vi "Data Analysis VI.vi"() -> ()   [LabVIEW 2022 SP3]
uses:
  0d05760f-8841-43ce-bf7e-76eea4fe5a42.vi
  <vilib>/Utility/file.llb/Read Delimited Spreadsheet (string).vi
  <vilib>/addons/Time Series Analysis/Statistical Analysis.llb/TSA Confidence Limits (Array).vi
  <vilib>/addons/Time Series Analysis/Statistical Analysis.llb/TSA Mean (Array).vi
  <vilib>/addons/Time Series Analysis/Series Preprocess.llb/TSA Moving Average (Array).vi
  <vilib>/addons/Time Series Analysis/Statistical Analysis.llb/TSA Vector Deviation and Variance (Waveform).vi
  <vilib>/addons/_Advanced Signal Processing/NI_AdvSigProcTSA.lvlib
  <vilib>/gmath/NI_Gmath.lvlib
  <vilib>/addons/Time Series Analysis/Series Preprocess.llb/TSA Moving Average (Waveform).vi
panel:
  in  "Which Days to Plot?":cluster{"Boolean":bool, "String":string}[](array[cluster])=[{"Boolean"=FALSE, "String"="Day 1"}, {"Boolean"=FALSE, "String"="Day 2"}, {"Boolean"=FALSE, "String"="Day 3"}, {"Boolean"=FALSE, "String"="Day 4"}, {"Boolean"=FALSE, "String"="Day 5"}]
  in  "What to Plot?":u16(ring) items=["X-Ray Tests (3 Days)", "Further Tests (5 Days)"]
  out "Calculate Temperature Change from Power Density - using formula described in Ekin.":cluster{dbl[], dbl[]}(graph)
  out "Voltage @ 1st Current Increment":cluster{dbl[], dbl[]}(graph)
  out "Dosage vs Ic":cluster{dbl[], dbl[]}(graph)
  out "decimated array 2":dbl[](array[numeric])
  out "decimated array":dbl[](array[numeric])
  out "Temperature Normaliser":cluster{dbl[], dbl[]}[](graph)
  out "Ic Power Law vs Time (COMPARE) 2":cluster{"Relative Times":dbl[], dbl[]}(graph)
  out "Array 3":path[](array[path])
  out "Array 2":path[](array[path])
  out "x = y?":bool
  out "Temperature vs Ic":T1(graph)
  in  "TempInterpolate Method":i32(ring)=2 items=["nearest", "linear", "spline", "cubic Hermite", "Lagrange"]
  in  "TempInterpolate Reverse Method":i32(ring)=2 items=["nearest", "linear", "spline", "cubic Hermite", "Lagrange"]
  out "Ic Temperature Curve of THEVA HTS Tape 2":cluster{"Temp Data":dbl[], "Ic Data":dbl[]}[](graph)
  out "NumPlots":i32
  out "Relative Times NaN'd":dbl[](array[numeric])
  out "Relative Times":dbl[](array[numeric])
  out "Dosage Characteristics":cluster{dbl[], dbl[]}[](graph)
  in  "Plot?":bool[](array[boolean])
  out "Concatenated Ic vs Time":cluster{dbl[], dbl[]}[](graph)
  out "Ic Power Law vs Time (COMPARE)":cluster{dbl[], dbl[]}[](graph)
  out "Historical Data 2":cluster{"Array":dbl[], "Array":dbl[]}[](graph)
  in  "(Baseline 1st)Shifted":dbl[](array[numeric])=[-200.4, -200.5] format="%#_13g"
  out "Expected Ic Fluctuation due to specified temperature range (A)":dbl[](array[numeric])
  out "percentage change":dbl[](array[numeric])
  out "Ic Temperature Curve of THEVA HTS Tape":cluster{"all rows":dbl[], "all rows":dbl[]}[](graph)
  out "Ic and Temperature vs Time":cluster{dbl[], dbl[]}[](graph)
  in  "length":i32=100
  in  "index":i32=20
  out "LogLog":cluster{dbl[], dbl[]}[](graph)
  out "error out":errorcluster
  out "Experimental Ic vs Temperature Corrected Ic":cluster{dbl[], dbl[]}[](graph)
  out "Absolute Ic Fluctuation":cluster{dbl[], dbl[]}(graph)
  out "Mean Run Temperature vs Time":cluster{dbl[], dbl[]}(graph)
  in  "Selected":dbl=10.0
  out "Different Model Comparisons for Selected Run":cluster{"Array":dbl[], "Array":dbl[]}[](graph)
  out "Compare Different Models vs TIME/DOSAGE":cluster{dbl[], dbl[]}[](graph)
  out "Total Dose over Measurement time (kGy)":dbl
  out "Maximum Dosage Rate (kGy/h)":dbl
  in  "Estimated Dose Rate 12cm from tube (Gy/s)":dbl=23.7
  out "Time vs Temperature":cluster{dbl[], dbl[]}(graph)
  out "Number of Runs":dbl
  out "Experiment Description":variant
  out "current time":timestamp
  in  "Array":path[](array[path])=[path "C:/Users/kumarr3/OneDrive - Victoria University of Wellington - STAFF/Documents/DataFiles/Xray runs/xray_FIRSTRUN", path "C:/Users/kumarr3/OneDrive - Victoria University of Wellington - STAFF/Documents/DataFiles/Xray runs/xray_secondrun_1902", path "C:/Users/kumarr3/OneDrive - Victoria University of Wellington - STAFF/Documents/DataFiles/Xray runs/xray_thirdrun_morning_2102", path "C:/Users/kumarr3/OneDrive - Victoria University of Wellington - STAFF/Documents/DataFiles/Copper Tests/Thursday_mixingtesting_01_voltmeter_alreadyON", path "C:/Users/kumarr3/OneDrive - Victoria University of Wellington - STAFF/Documents/DataFiles/Copper Tests/Thursday_mixingtesting_01_voltmeter_alreadyON", path "C:/Users/kumarr3/OneDrive - Victoria University of Wellington - STAFF/Documents/DataFiles/Copper Tests/Friday_mixingtest_voltmeter_justturnedon", path "C:/Users/kumarr3/OneDrive - Victoria University of Wellington - STAFF/Documents/DataFiles/Copper Tests/Monday_mixingtest_voltmeterONallweekend", path "C:/Users/kumarr3/OneDrive - Victoria University of Wellington - STAFF/Documents/DataFiles/Copper Tests/Tuesday_bothmeters_onovernight"] caption="Load File Path or Directory"
  # "Data extracted from tdms file, plotted against TIME/DOSAGE"
  # "Temperature Correction Analysis"
  # "Loading Information"
  # "Temperature Interpolation"
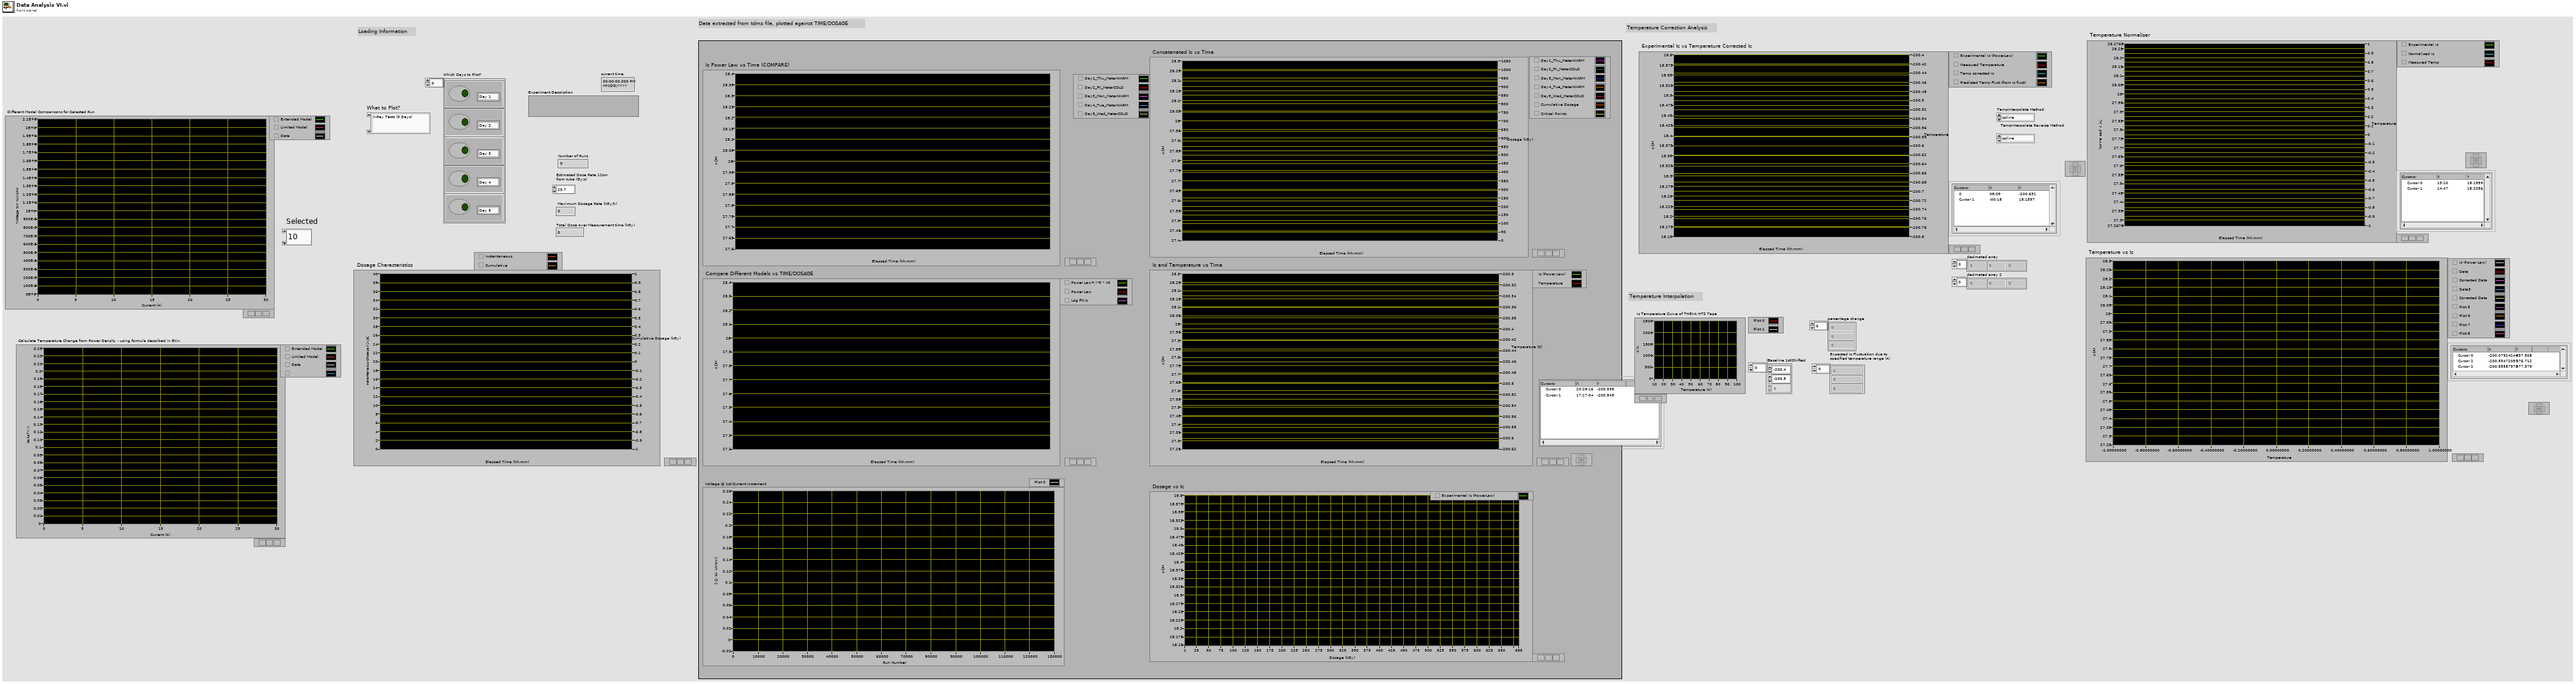
[diagram p1: front panel]
types:
  T1 = cluster{"Ic array (Power Law)":dbl[], "Mean Temp Array":dbl[]}[]
  T2 = cluster{"Dosage RelTimes":dbl[], "Cumul Dosages":dbl[], "Instantaneous Dosages":dbl[]}
  T3 = cluster{"Mean Temp Array":dbl[], "Lower Temp Array":dbl[], "Upper Temp Array":dbl[]}
  T4 = cluster{"Ic Array (Extnded)":dbl[], "Ic array (Power Law)":dbl[], "Relative Times":dbl[], "LogLog FIt":dbl[], "Absolute Ic Fluctuation":dbl[], "Temp Corrected Data":dbl[], "Upper Corrected":dbl[], "Lower Corrected":dbl[], "Smoothed Power Law":dbl[]}
  T5 = cluster{"I indexed":dbl[], "Best Linear Fit":dbl[]}
  T6 = cluster{"I indexed":dbl[], "Best Linear Fit":dbl[]}[]
  T7 = cluster{"Relative Times":dbl[], "Ic Array (Extnded)":dbl[]}
  T8 = cluster{"Relative Times":dbl[], "Ic Array (Extnded)":dbl[]}[]
  T9 = cluster{"Instant. Dos. Times":dbl[], "Instant. Dosages":dbl[]}
  T10 = cluster{"Cumul Dos. Times":dbl[], "Cumul Dosages":dbl[]}
  T11 = cluster{"Cumul Dos. Times":dbl[], "Cumul Dosages":dbl[]}[]
  T12 = cluster{"Critical Times":dbl[], "Critical Dosages":dbl[]}
  T13 = cluster{"Mean Temp Array":dbl[], "Ic array (Power Law)":dbl[]}
  T14 = cluster{"Predicted Temp (C)":dbl[], "xi used":dbl[]}
  T15 = cluster{"Relative Times NaN'd":dbl[], "Corrected Ic":dbl[]}
  T16 = cluster{"Predicted Temp (C)":dbl[], "xi used":dbl[]}[]
  T17 = cluster{"Mean Temp Array":dbl[], "Corrected Ic":dbl[]}[]
  T18 = cluster{"Relative Times NaN'd":dbl[], "Predicted Temp (C)":dbl[]}
  T19 = cluster{"Critical Times":dbl[], "Critical Dosages":dbl[]}[]
  T20 = cluster{"Relative Times NaN'd":dbl[], "Predicted Temp (C)":dbl[]}[]
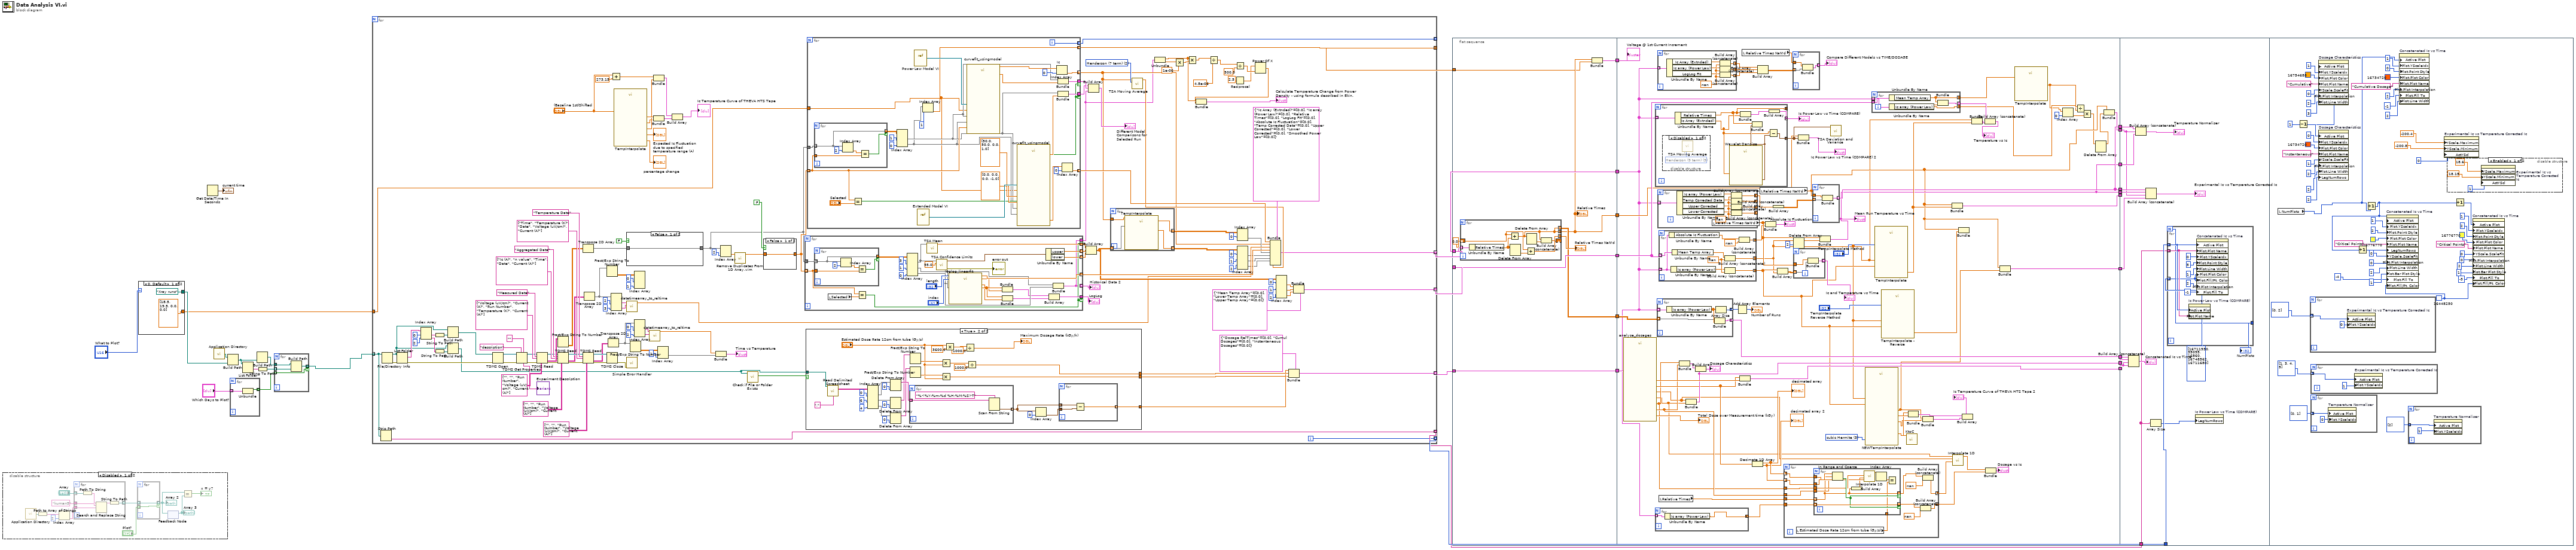
[diagram p0: block diagram]
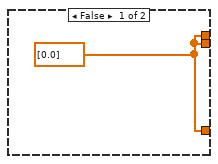
[diagram p2: hidden frame]
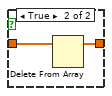
[diagram p3: hidden frame]
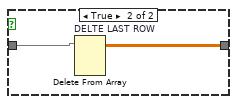
[diagram p4: hidden frame]
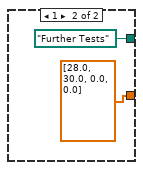
[diagram p6: hidden frame]
diagram:
  n1 = disable-structure shown="Disabled" {
    frame Disabled {
      n2 = call <vilib>:"Application Directory.vi"() -> ("Application Directory"=w41:path)
      n3 = Path to Array of Strings(0:w41) -> (2:w42:string[])  [unwired: 1 out]
      n4 = Index Array(array=w42, index=2) -> (element=w43:string)
      n5 = for {
        tunnel: "Array" -> [w51] mode=indexing
        tunnel: w43 -> [w49]
        tunnel: "kumarr3" ("search string") -> [w48]
        tunnel: [w46] -> w45 mode=indexing
        n6 = Path To String(path=w51) -> (string=w50:string)
        n7 = Search and Replace String(input string=w50, search string=w48, replace string=w49) -> (result string=w47:string)  [unwired: 5 in, 3 out]
        n8 = String To Path(string=w47) -> (path=w46:path)
      }
      n9 = for {
        tunnel: [w53] -> w39 mode=indexing if=w52
        tunnel: w45 -> [w53] mode=indexing
        tunnel: "Plot?" -> [w52] mode=indexing
      }
      "Array 2" <- w39
      n10 = feedback #1() -> (w38:path[])  [unwired: 1 in]
      "Array 3" <- w38
      n11 = feedback-in #1(w39) -> ()
      n12 = Equal?(x=w39, y=w38) -> (x = y?=→"x = y?":bool)
    }
    frame Enabled {
    }
  }
  n13 = case shown="0, Default" "What to Plot?" {
    tunnel: [path "Xray runs" path "Further Tests"] -> w9
    tunnel: [dbl[] [18.5, 19.5, 0.0, 0.0] dbl[] [28.0, 30.0, 0.0, 0.0]] -> w1
    frame 0, Default {
    }
    frame 1 {
    }
  }
  n14 = Get Date/Time In Seconds() -> (seconds since 1Jan1904=→"current time":timestamp)
  n15 = call <vilib>:"Application Directory.vi"() -> ("Application Directory"=w8:path)
  n16 = Build Path(base path=w8, name or relative path=w9) -> (appended path=w6:path)
  n17 = for {
    tunnel: "Which Days to Plot?" -> [w59] mode=indexing
    tunnel: [w58] -> w4 mode=indexing
    n18 = Unbundle(w59) -> ("Boolean"=w58:bool)  [unwired: 1 out]
  }
  n19 = List Folder(path=w6) -> (folder names=w7:string[])  [unwired: 3 in, 3 out]
  n20 = Build Path(name or relative path=w6) -> (appended path=w3:path)  [unwired: 1 in]
  n21 = String To Path(string=w7) -> (path=w5:path[])
  n22 = for {
    tunnel: [w60] -> w2 mode=indexing if=w63
    tunnel: w5 -> [w61] mode=indexing
    tunnel: w4 -> [w63] mode=indexing
    tunnel: w3 -> [w62]
    n23 = Build Path(base path=w62, name or relative path=w61) -> (appended path=w60:path)
  }
  n24 = for {
    tunnel: w2 -> [w140] mode=indexing
    tunnel: [w85] -> w22 mode=indexing
    tunnel: [w84] -> w21 mode=indexing
    tunnel: [w83] -> w20 mode=indexing
    tunnel: [w107] -> w19 mode=indexing
    tunnel: [w106] -> w18 mode=indexing
    tunnel: [w80] -> _ mode=indexing
    tunnel: [w79] -> w13 mode=concatenating
    tunnel: w1 -> [w64]
    i -> [w107]
    w97 = 2 items=["Spencer (15 term)"=1, "Henderson (7 term)"=2, "Henderson (9 term)"=3, "Henderson (13 term)"=4, "Henderson (23 term)"=5] ("method")
    n25 = Strip Path(path=w140) -> (name=w106:string)  [unwired: 1 out]
    n26 = File/Directory Info(path=w140) -> (path out=w113:path, error out=w200:errorcluster)  [unwired: 1 in, 5 out]
    n27 = List Folder(path=w113, error in=w200) -> (filenames=w138:string[], error out=w198:errorcluster)  [unwired: 2 in, 2 out]
    n28 = Index Array(array=w138, index #1=0 ("index"), index #2=2 ("index")) -> (element #1=w139:string, element #2=w114:string)
    n29 = String To Path(string=w139) -> (path=w197:path)
    n30 = String To Path(string=w114) -> (path=w112:path)
    n31 = Build Path(base path=w113, name or relative path=w197) -> (appended path=w157:path)
    n32 = Build Path(base path=w113, name or relative path=w112) -> (appended path=w81:path)
    n33 = TDMS Open(8:w198, 11:w157) -> (0:w186:errorcluster, 3:w187:refnum<k34>)  [unwired: 5 in]
    n34 = TDMS Get Properties(5:"", 7:"description", 8:w186, 11:w187) -> (0:w184:errorcluster, 3:w185:refnum<k34>, 4:→"Experiment Description":string)  [unwired: 2 in, 3 out]
    n35 = TDMS Read(0:w185, 5:"Measured Data" ("group name in"), 7:string[] ["Voltage (uV/cm)", "Current (A)", "Run Number", "Temperature (K)", "Current (A)"] ("channel name(s) in (Untitled)"), 11:w184, 12:string[][] [["", "", "Run Number", "Voltage (uV/cm)", "Current (A)"]] ("channel name(s) in (Untitled)")) -> (4:w174:refnum<k34>, 10:w193:string[][], 15:w173:errorcluster)  [unwired: 3 in, 3 out]
    n36 = Fract/Exp String To Number(string=w193) -> (number=w156:dbl[][])  [unwired: 3 in, 1 out]
    n37 = TDMS Read(0:w174, 5:"Aggregated Data" ("group name in"), 7:string[] ["Ic (A)", "n value", "Time", "Date", "Current (A)"] ("channel name(s) in (Untitled)"), 11:w173, 12:string[][] [["", "", "Run Number", "Voltage (uV/cm)", "Current (A)"]] ("channel name(s) in (Untitled)")) -> (4:w172:refnum<k34>, 10:w166:string[][], 15:w171:errorcluster)  [unwired: 3 in, 3 out]
    n38 = TDMS Read(0:w172, 5:"Temperature Data" ("group name in"), 7:string[] ["Time", "Temperature (K)", "Date", "Voltage (uV/cm)", "Current (A)"] ("channel name(s) in (Untitled)"), 11:w171, 12:string[][] [["", "", "Run Number", "Voltage (uV/cm)", "Current (A)"]] ("channel name(s) in (Untitled)")) -> (4:w176:refnum<k34>, 10:w169:string[][], 15:w175:errorcluster)  [unwired: 3 in, 3 out]
    n39 = Transpose 2D Array(2D array=w156) -> (transposed array=w155:dbl[][])
    n40 = Transpose 2D Array(2D array=w166) -> (transposed array=w141:string[][])
    n41 = Fract/Exp String To Number(string=w141) -> (number=w165:dbl[][])  [unwired: 3 in, 1 out]
    n42 = TDMS Close(8:w175, 11:w176) -> (0:w180:errorcluster)  [unwired: 1 out]
    n43 = Transpose 2D Array(2D array=w169) -> (transposed array=w151:string[][])
    n44 = Add(x="(Baseline 1st)Shifted", y=273.15) -> (x+y=w91:dbl[])
    n45 = Index Array(array=w141, index (col) #1=2 ("disabled index (col)"), index (col) #2=3 ("index (col)")) -> (element #1=w150:string[], element #2=w122:string[])  [unwired: 2 in]
    n46 = call "TempInterpolate.vi"("(Baseline 1st) Shifted"="(Baseline 1st)Shifted") -> ("Temp Data"=w95:dbl[], "Ic Data"=w87:dbl[], "Ic Fluct (from baseline)"=→"Expected Ic Fluctuation due to specified temperature range (A)":dbl[], "percentage change"=→"percentage change":dbl[], "Raw Interpolated Ic"=w93:dbl[])  [unwired: 5 in, 1 out]
    n47 = case shown="False" FALSE {
      tunnel: w155 -> [w273 w275]
      tunnel: [w273 w274] -> w145
      frame False {
      }
      frame True {
        n48 = Delete From Array "DELTE LAST ROW"(array=w275) -> (array with subset deleted=w274:dbl[][])  [unwired: 3 in, 1 out]
      }
    }
    n49 = call "datetimearray_to_reltime.vi"("Date Array"=w122, "Time Array"=w150) -> ("Rel. time array"=w109:dbl[])  [unwired: 9 in]
    n50 = call <vilib>:"Simple Error Handler.vi"("error in (no error)"=w180) -> ()  [unwired: 2 in, 7 out]
    n51 = Fract/Exp String To Number(string=w151) -> (number=w168:dbl[][])  [unwired: 3 in, 1 out]
    n52 = Index Array(array=w165, index (col) #1=0 ("disabled index (col)"), index (col) #2=1 ("index (col)")) -> ()  [unwired: 2 in, 2 out]
    n53 = Index Array(array=w151, index (col) #1=0 ("disabled index (col)"), index (col) #2=2 ("index (col)")) -> (element #1=w154:string[], element #2=w119:string[])  [unwired: 2 in]
    n54 = call "datetimearray_to_reltime.vi"("Date Array"=w119, "Time Array"=w154) -> ("Rel. time array"=w153:dbl[])  [unwired: 9 in]
    n55 = Bundle(w91, "Raw Interpolated Ic"=w93) -> (w89:cluster{dbl[], "Raw Interpolated Ic":dbl[]})  [unwired: 1 in]
    n56 = Bundle("Temp Data"=w95, "Ic Data"=w87) -> (w88:cluster{"Temp Data":dbl[], "Ic Data":dbl[]})  [unwired: 1 in]
    n57 = Index Array(array=w168, index (col)=1 ("disabled index (col)")) -> (element=w161:dbl[])  [unwired: 1 in]
    n58 = Build Array(w89, w88) -> (→"Ic Temperature Curve of THEVA HTS Tape":cluster{"Temp Data":dbl[], "Ic Data":dbl[]}[])
    n59 = Bundle("Rel. time array"=w153, w161) -> (→"Time vs Temperature":cluster{"Rel. time array":dbl[], dbl[]})  [unwired: 1 in]
    n60 = Index Array(array=w145, index (col)=2 ("disabled index (col)")) -> (element=w160:dbl[])  [unwired: 1 in]
    n61 = call "Remove Duplicates From 1D Array.vim"("array"=w160) -> ("array with duplicates removed"=w148:dbl[])  [unwired: 10 in]
    n62 = call <vilib>:"Check if File or Folder Exists.vi"("path"=w81) -> ("file or folder exists?"=w82:bool)  [unwired: 8 in, 2 out]
    n63 = case shown="False" FALSE {
      tunnel: w148 -> [w270 w272]
      tunnel: [w270 w271] -> w146
      frame False {
      }
      frame True {
        n64 = Delete From Array(array=w272) -> (array with subset deleted=w271:dbl[])  [unwired: 2 in, 1 out]
      }
    }
    n65 = for {
      tunnel: w145 -> [w264]
      tunnel: w146 -> [w255] mode=indexing
      tunnel: [w239] -> w78 if=w241
      tunnel: [w263] -> w136 mode=indexing
      tunnel: [w258] -> w143 mode=indexing
      tunnel: [w257] -> w142 mode=indexing
      tunnel: [w256] -> w144 mode=indexing
      tunnel: [w242] -> w117 if=w241
      tunnel: [w239] -> w116 mode=indexing
      n66 = for {
        tunnel: w264 -> [w267] mode=indexing
        tunnel: [w267] -> w253 mode=indexing if=w266
        tunnel: w255 -> [w265]
        n67 = Index Array(array=w267, index=2) -> (element=w268:dbl)
        n68 = Equal?(x=w268, y=w265) -> (x = y?=w266:bool)
      }
      n69 = local read "Selected"() -> (w238:dbl)
      n70 = Equal?(x=w255, y=w238) -> (x = y?=w241:bool)
      n71 = Index Array(array=w253, index (col) #1=3 ("disabled index (col)"), index (col) #2=1 ("index (col)"), index (col) #3=0 ("index (col)")) -> (element #1=w259:dbl[], element #2=w248:dbl[], element #3=w247:dbl[])  [unwired: 3 in]
      n72 = call-poly <vilib>:"TSA Mean.vi"("Xt"=w259) -> ("mean"=w256:dbl)  [unwired: 9 in, 1 out]
      n73 = call-poly <vilib>:"TSA Confidence Limits.vi"("confidence level (%)"=95.0, "Xt"=w259) -> ("error out"=→"error out":errorcluster, "mean limits"=w261:cluster{"upper":dbl, "lower":dbl})  [unwired: 7 in, 1 out]
      n74 = call "loglog_linearfit.vi"("Current"=w248, "Voltage"=w247, "index"="index", "length"="length") -> ("Best Linear Fit"=w245:dbl[], "V indexed"=w240:dbl[], "Ic"=w263:dbl, "I indexed"=w246:dbl[])  [unwired: 3 in, 1 out]
      n75 = Bundle("I indexed"=w246, "V indexed"=w240) -> (w244:cluster{"I indexed":dbl[], "V indexed":dbl[]})  [unwired: 1 in]
      n76 = Bundle("I indexed"=w246, "Best Linear Fit"=w245) -> (w243:T5)  [unwired: 1 in]
      n77 = Unbundle By Name(w261) -> ("upper"=w258:dbl, "lower"=w257:dbl)
      n78 = Build Array(w244, w243) -> (w242:T6)
      n79 = Bundle(w248, w247) -> (w239:cluster{dbl[], dbl[]})  [unwired: 1 in]
    }
    "LogLog" <- w117
    "Historical Data 2" <- w116
    n80 = case shown="True" w82 {
      tunnel: w81 -> [_ w224]
      tunnel: [w201 w210] -> w110
      tunnel: [w201 w209] -> w108
      tunnel: [w201 w205] -> w104
      frame False {
        w201 = dbl[] [0.0]
      }
      frame True {
        n81 = call-poly <vilib>:"Read Delimited Spreadsheet.vi"("file path (dialog if empty)"=w224, "delimiter (\\t)"="," ("delimiter (\\t)")) -> ("all rows"=w227:string[][])  [unwired: 8 in, 5 out]
        n82 = Index Array(array=w227, index (col) #1=0 ("disabled index (col)"), index (col) #2=6 ("index (col)"), index (col) #3=4 ("index (col)")) -> (element #1=w220:string[], element #2=w212:string[], element #3=w203:string[])  [unwired: 3 in]
        n83 = Delete From Array(array=w220, index=0) -> (array with subset deleted=w218:string[])  [unwired: 1 in, 1 out]
        n84 = Delete From Array(array=w212, index=0) -> (array with subset deleted=w211:string[])  [unwired: 1 in, 1 out]
        n85 = Delete From Array(array=w203, index=0) -> (array with subset deleted=w202:string[])  [unwired: 1 in, 1 out]
        n86 = for {
          tunnel: [w236] -> w223 mode=indexing
          tunnel: w218 -> [w235] mode=indexing
          n87 = Scan From String(format string="%<%Y-%m-%d %H:%M:%S>T" ("time format string (%c)"), input string=w235) -> (output 1=w236:timestamp)  [unwired: 3 in, 3 out]
        }
        n88 = Fract/Exp String To Number(string=w211) -> (number=w214:dbl[])  [unwired: 3 in, 1 out]
        n89 = Fract/Exp String To Number(string=w202) -> (number=w207:dbl[])  [unwired: 3 in, 1 out]
        n90 = Multiply(x=w214, y="Estimated Dose Rate 12cm from tube (Gy/s)") -> (x*y=w215:dbl[])
        n91 = Multiply(x=w207, y="Estimated Dose Rate 12cm from tube (Gy/s)") -> (x*y=w205:dbl[])
        n92 = Multiply(x="Estimated Dose Rate 12cm from tube (Gy/s)", y=3600.0) -> (x*y=w230:dbl)
        n93 = Divide(x=w230, y=1000.0) -> (x/y=→"Maximum Dosage Rate (kGy/h)":dbl)
        n94 = Divide(x=w215, y=1000.0) -> (x/y=w210:dbl[])
        n95 = Index Array(array=w223, index=0 ("disabled index (col)")) -> (element=w222:timestamp)
        n96 = for {
          tunnel: w223 -> [w233] mode=indexing
          tunnel: w222 -> [w234]
          tunnel: [w232] -> w209 mode=indexing
          n97 = Subtract(x=w233, y=w234) -> (x-y=w232:dbl)
        }
      }
    }
    n98 = for {
      tunnel: w145 -> [w306]
      tunnel: w146 -> [w299] mode=indexing
      tunnel: [w304] -> w158 if=w287
      tunnel: [w301] -> w86 mode=indexing
      tunnel: [w288] -> w118 if=w287
      tunnel: [w286] -> w105 mode=indexing
      tunnel: [w283] -> w79 mode=indexing
      tunnel: [w282] -> w80 mode=indexing
      tunnel: w64 -> [w280]
      i -> [w282]
      n99 = for {
        tunnel: w306 -> [w309] mode=indexing
        tunnel: [w309] -> w290 mode=indexing if=w308
        tunnel: w299 -> [w307]
        n100 = Index Array(array=w309, index=2) -> (element=w310:dbl)
        n101 = Equal?(x=w310, y=w307) -> (x = y?=w308:bool)
      }
      n102 = Equal?(x=w299, y="Selected") -> (x = y?=w287:bool)
      n103 = Index Array(array=w290, index (col) #1=1 ("disabled index (col)"), index (col) #2=0 ("index (col)")) -> (element #1=w285:dbl[], element #2=w281:dbl[])  [unwired: 2 in]
      n104 = vi-ref "Power Law Model VI.vi"() -> (w298:refnum<vi>)
      n105 = vi-ref "Extended Model VI.vi"() -> (w296:refnum<vi>)
      n106 = Index Array(array=w281, index=1) -> (element=w283:dbl)
      n107 = call "curvefit_usingmodel.vi"("Y"=w281, "initial parameters"=w280, "Run Number"=w299, "X"=w285, "model"=w298) -> ("Fitted Curve"=w305:dbl[], "best fit parameters"=w303:dbl[])  [unwired: 3 in, 2 out]
      n108 = call "curvefit_usingmodel.vi"("Y"=w281, "initial parameters"=w280, "param upper bounds"=dbl[] [0.0, 0.0, 0.0, -1.0], "X"=w285, "param lower bounds"=dbl[] [50.0, 50.0, 0.0, 1.0], "model"=w296) -> ("Fitted Curve"=w289:dbl[], "best fit parameters"=w293:dbl[])  [unwired: 2 in, 2 out]
      n109 = Index Array "Ic"(array=w303, index=0 ("index (col)")) -> (element=w301:dbl)
      n110 = Bundle(w285, "Fitted Curve"=w305) -> (w304:cluster{dbl[], "Fitted Curve":dbl[]})  [unwired: 1 in]
      n111 = Bundle(w285, "Fitted Curve"=w289) -> (w288:cluster{dbl[], "Fitted Curve":dbl[]})  [unwired: 1 in]
      n112 = Index Array(array=w293, index=0 ("index (col)")) -> (element=w286:dbl)
    }
    n113 = Build Array(w144, w143, w142) -> (w126:dbl[][])
    n114 = Build Array(w118, w158, w78) -> (→"Different Model Comparisons for Selected Run":cluster{dbl[], "Fitted Curve":dbl[]}[])
    n115 = for {
      tunnel: w126 -> [w278] mode=indexing
      tunnel: w86 -> [w279]
      tunnel: [w277] -> w135 mode=indexing
      tunnel: [w276] -> w124 mode=indexing
      n116 = call "TempInterpolate.vi"("(Baseline 1st) Shifted"=w278, "True Experimental Data"=w279) -> ("Ic Fluct (from baseline)"=w276:dbl[], "Corrected Ic"=w277:dbl[])  [unwired: 4 in, 4 out]
    }
    n117 = call-poly <vilib>:"TSA Moving Average.vi"("method"=w97, "Xt"=w86) -> ("Xt out"=w96:dbl[])  [unwired: 8 in, 1 out]
    n118 = Unbundle(w78) -> (w72:dbl[], w77:dbl[])
    n119 = Multiply(x=w77, y=1e-06) -> (x*y=w75:dbl[])
    n120 = Multiply(x=w72, y=w75) -> (x*y=w74:dbl[])
    n121 = Divide(x=w74, y=4.8e-06) -> (x/y=w71:dbl[])
    n122 = Reciprocal(x=2.5 ("y")) -> (1/x=w67:dbl)
    n123 = Divide(x=w71, y=500.0) -> (x/y=w68:dbl[])
    n124 = Index Array(array=w124, index (row)=0) -> (element=w100:dbl[])  [unwired: 1 in]
    n125 = Index Array(array=w135, index (row) #1=0 ("index (row)"), index (row) #2=1 ("index (row)"), index (row) #3=2 ("index (row)")) -> (element #1=w101:dbl[], element #2=w99:dbl[], element #3=w98:dbl[])  [unwired: 3 in]
    n126 = Power Of X(1:w68, 2:w67) -> (0:w66:dbl[])
    n127 = Bundle(w72, w66) -> (→"Calculate Temperature Change from Power Density - using formula described in Ekin.":cluster{dbl[], dbl[]})  [unwired: 1 in]
    n128 = Bundle(cluster=T4 {"Ic Array (Extnded)"=[0.0], "Ic array (Power Law)"=[0.0], "Relative Times"=[0.0], "LogLog FIt"=[0.0], "Absolute Ic Fluctuation"=[0.0], "Temp Corrected Data"=[0.0], "Upper Corrected"=[0.0], "Lower Corrected"=[0.0], "Smoothed Power Law"=[0.0]} ("input cluster"), "Ic Array (Extnded)"=w105, "Ic array (Power Law)"=w86, "Relative Times"=w109, "LogLog FIt"=w136, "Absolute Ic Fluctuation"=w100, "Temp Corrected Data"=w101, "Upper Corrected"=w99, "Lower Corrected"=w98, "Smoothed Power Law"=w96) -> (w85:T4)
    n129 = Index Array(array=w126, index (row) #1=0 ("index (row)"), index (row) #2=1 ("index (row)"), index (row) #3=2 ("index (row)")) -> (element #1=w129:dbl[], element #2=w128:dbl[], element #3=w127:dbl[])  [unwired: 3 in]
    n130 = Bundle(cluster=T2 {"Dosage RelTimes"=[0.0], "Cumul Dosages"=[0.0], "Instantaneous Dosages"=[0.0]} ("input cluster"), "Dosage RelTimes"=w108, "Cumul Dosages"=w110, "Instantaneous Dosages"=w104) -> (w83:T2)
    n131 = Bundle(cluster=T3 {"Mean Temp Array"=[0.0], "Lower Temp Array"=[0.0], "Upper Temp Array"=[0.0]} ("input cluster"), "Mean Temp Array"=w129, "Lower Temp Array"=w128, "Upper Temp Array"=w127) -> (w84:T3)
  }
  n132 = flat-sequence {
    tunnel: w22 -> [w316]
    tunnel: [w314] -> w33
    tunnel: [w315] -> w32
    tunnel: [w316] -> w31
    tunnel: w21 -> [w319]
    tunnel: [w319] -> w30
    tunnel: w20 -> [w317]
    tunnel: [w317] -> w23
    tunnel: w13 -> [w313]
    tunnel: [w312] -> w12
    tunnel: w33 -> [w359]
    tunnel: w32 -> [w397]
    tunnel: w31 -> [w340]
    tunnel: w30 -> [w378]
    tunnel: [w355] -> w29
    tunnel: [w350] -> w28
    tunnel: [w394] -> w27
    tunnel: [w395] -> w26
    tunnel: [w388] -> w25
    tunnel: [w389] -> w24
    tunnel: w23 -> [w387]
    tunnel: [w364] -> w17
    tunnel: [w355] -> w16
    tunnel: [w353] -> w15
    tunnel: [w350] -> w14
    tunnel: w12 -> [w329]
    tunnel: w29 -> [w503]
    tunnel: w28 -> [w502]
    tunnel: w27 -> [_]
    tunnel: w26 -> [w500]
    tunnel: w25 -> [w499]
    tunnel: w24 -> [w498]
    tunnel: w19 -> [w496]
    tunnel: w18 -> [w489]
    tunnel: w17 -> [w494]
    tunnel: w16 -> [w492]
    tunnel: w15 -> [w490]
    tunnel: w14 -> [w491]
    frame #0 {
      n133 = for {
        tunnel: w316 -> [w326] mode=indexing
        shift-right: [w324] -> _
        shift-left: 0.0 -> [w325]
        tunnel: [w321] -> w314 mode=concatenating
        tunnel: [w322] -> w320 mode=concatenating
        tunnel: [w321] -> w315 mode=indexing
        n134 = Unbundle By Name(w326) -> ("Relative Times"=w327:dbl[])
        n135 = Add(x=w325, y=w327) -> (x+y=w321:dbl[])
        n136 = Delete From Array(array=w327) -> (deleted portion=w328:dbl)  [unwired: 2 in, 1 out]
        n137 = Add(x=w325, y=w328) -> (x+y=w324:dbl)
        n138 = Delete From Array(array=w321) -> (deleted portion=w323:dbl)  [unwired: 2 in, 1 out]
        n139 = Build Array (concatenate)(w321, w323) -> (w322:dbl[])
      }
      "Relative Times" <- w314
      "Relative Times NaN'd" <- w320
      n140 = Bundle(w314, w313) -> (w312:cluster{dbl[], dbl[]})  [unwired: 1 in]
    }
    frame #1 {
      w367 = 3 items=["nearest", "linear", "spline", "cubic Hermite", "Lagrange"] ("method")
      n141 = call "analyse_dosages.vi"("Dosage Cluster"=w387) -> ("Cumul Dosages"=w334:dbl[], "Cumul Dos. Times"=w335:dbl[], "Instant. Dos. Times"=w336:dbl[], "Critical Times"=w343:dbl[], "Instant. Dosages"=w337:dbl[], "Critical Dosages"=w390:dbl[], "Total Dosage (kGy)"=→"Total Dose over Measurement time (kGy)":dbl)  [unwired: 4 in]
      n142 = for {
        tunnel: w340 -> [w408] mode=indexing
        tunnel: [w407] -> w339 mode=concatenating
        n143 = Unbundle By Name(w408) -> ("Ic array (Power Law)"=w407:dbl[])
      }
      n144 = for {
        tunnel: w340 -> [w444] mode=indexing
        tunnel: [w442] -> w386 mode=concatenating
        tunnel: [w441] -> w360 mode=concatenating
        tunnel: [w440] -> _ mode=concatenating
        n145 = disable-structure shown="Disabled" {
          frame Disabled {
            w445 = 3 items=["Spencer (15 term)"=1, "Henderson (7 term)"=2, "Henderson (9 term)"=3, "Henderson (13 term)"=4, "Henderson (23 term)"=5] ("method")
            n146 = call-poly <vilib>:"TSA Moving Average.vi"("method"=w445) -> ()  [unwired: 9 in, 2 out]
          }
          frame Enabled {
          }
        }
        n147 = Unbundle By Name(w444) -> ("Relative Times"=w440:dbl[], "Ic Array (Extnded)"=w438:dbl[])
        n148 = call "Wavelet Denoise"("Signal"=w438) -> ("Denoised Signal"=w439:waveform(dbl))  [unwired: 9 in, 1 out]
        n149 = Bundle("Relative Times"=w440, "Ic Array (Extnded)"=w438) -> (w443:T7)  [unwired: 1 in]
        n150 = Bundle("Relative Times"=w440, "Denoised Signal"=w439) -> ()  [unwired: 1 in, 1 out]
        n151 = Subtract(x=w438, y=w439) -> (x-y=w441:waveform(dbl)[])
        n152 = Build Array(w443) -> (w442:T8)
      }
      "Ic Power Law vs Time (COMPARE)" <- w386
      n153 = for {
        tunnel: w397 -> [w447] mode=indexing
        tunnel: w340 -> [w450] mode=indexing
        tunnel: [w448] -> w396 mode=indexing
        tunnel: [w446] -> w395 mode=indexing
        n154 = Unbundle By Name(w450) -> ("Ic array (Power Law)"=w449:dbl[])
        n155 = Bundle(w447, "Ic array (Power Law)"=w449) -> (w446:cluster{dbl[], "Ic array (Power Law)":dbl[]})  [unwired: 1 in]
        n156 = Array Size(array=w449) -> (size(s)=w448:i32)
      }
      n157 = for {
        tunnel: [w454] -> w363 mode=concatenating
        tunnel: [w453] -> w361 mode=concatenating
        tunnel: [w452] -> w399 mode=concatenating
        tunnel: w340 -> [w451] mode=indexing
        w458 = nan ("element")
        n158 = Unbundle By Name(w451) -> ("Ic Array (Extnded)"=w457:dbl[], "Ic array (Power Law)"=w456:dbl[], "LogLog FIt"=w455:dbl[])
        n159 = Build Array (concatenate)(w457, w458) -> (w454:dbl[])
        n160 = Build Array (concatenate)(w456, w458) -> (w453:dbl[])
        n161 = Build Array (concatenate)(w455, w458) -> (w452:dbl[])
      }
      n162 = for {
        tunnel: w340 -> [w483] mode=indexing
        tunnel: [w485] -> w385 mode=concatenating
        tunnel: [w484] -> _ mode=concatenating
        tunnel: [w479] -> _ mode=concatenating
        tunnel: [w478] -> _ mode=concatenating
        w482 = nan ("element")
        n163 = Unbundle By Name(w483) -> ("Ic array (Power Law)"=w487:dbl[], "Temp Corrected Data"=w486:dbl[], "Upper Corrected"=w481:dbl[], "Lower Corrected"=w480:dbl[])
        n164 = Build Array (concatenate)(w487, w482) -> (w485:dbl[])
        n165 = Build Array (concatenate)(w486, w482) -> (w484:dbl[])
        n166 = Build Array (concatenate)(w481, w482) -> (w479:dbl[])
        n167 = Build Array (concatenate)(w480, w482) -> (w478:dbl[])
      }
      n168 = for {
        tunnel: [w463] -> w379 mode=concatenating
        tunnel: [w462] -> w366 mode=concatenating
        tunnel: [w461] -> w346 mode=concatenating
        tunnel: w378 -> [w460] mode=indexing
        tunnel: w340 -> [w459] mode=indexing
        w467 = nan ("array")
        n169 = Unbundle By Name(w459) -> ("Absolute Ic Fluctuation"=w465:dbl[])
        n170 = Unbundle By Name(w459) -> ("Ic array (Power Law)"=w466:dbl[])
        n171 = Unbundle By Name(w460) -> ("Mean Temp Array"=w468:dbl[])
        n172 = Build Array (concatenate)(w468, w467) -> (w461:dbl[])
        n173 = Build Array (concatenate)(w466, w467) -> (w462:dbl[])
        n174 = Build Array (concatenate)(w465, nan ("array")) -> (w463:dbl[])
      }
      n175 = local read "Relative Times"() -> (w338:dbl[])
      n176 = Bundle("Instant. Dos. Times"=w336, "Instant. Dosages"=w337) -> (w393:T9)  [unwired: 1 in]
      n177 = Bundle("Cumul Dos. Times"=w335, "Cumul Dosages"=w334) -> (w388:T10)  [unwired: 1 in]
      n178 = Build Array(w393, w388) -> (→"Dosage Characteristics":T11)
      n179 = local read "Relative Times NaN'd"() -> (w400:dbl[])
      n180 = Add Array Elements(numeric array=w396) -> (sum=→"Number of Runs":i32)
      n181 = Bundle("Critical Times"=w343, "Critical Dosages"=w390) -> (w389:T12)  [unwired: 1 in]
      n182 = local read "Relative Times NaN'd"() -> (w398:dbl[])
      n183 = Decimate 1D Array(w343) -> (w342:dbl[], w341:dbl[])
      "decimated array" <- w342
      "decimated array 2" <- w341
      n184 = Build Array(w363, w361, w399) -> (w401:dbl[][])
      n185 = local read "Relative Times NaN'd"() -> (w349:dbl[])
      n186 = Bundle("Relative Times NaN'd"=w400, w379) -> (→"Absolute Ic Fluctuation":cluster{"Relative Times NaN'd":dbl[], dbl[]})  [unwired: 1 in]
      n187 = Build Array(w385) -> (w403:dbl[][])
      n188 = Build Array(w366, w346) -> (w404:dbl[][])
      n189 = for {
        tunnel: w342 -> [w419] mode=indexing
        tunnel: w341 -> [w418] mode=indexing
        tunnel: w339 -> [w420]
        tunnel: w338 -> [w421]
        tunnel: [w409] -> w333 mode=concatenating
        tunnel: [w412] -> w330 mode=concatenating
        tunnel: w337 -> [w417]
        tunnel: w336 -> [w416]
        n190 = local read "Estimated Dose Rate 12cm from tube (Gy/s)"() -> (w415:dbl)
        n191 = for {
          tunnel: w421 -> [w425] mode=indexing
          tunnel: w420 -> [w430] mode=indexing
          tunnel: w419 -> [w432]
          tunnel: w418 -> [w431]
          tunnel: [w425] -> w410 mode=indexing if=w429
          tunnel: [w430] -> w413 mode=indexing if=w429
          tunnel: w417 -> [w427]
          tunnel: w416 -> [w428]
          tunnel: w415 -> [w422]
          n192 = In Range and Coerce(upper limit=w431, x=w425, lower limit=w432) -> (In Range?=w429:bool)  [unwired: 1 out]
          n193 = Build Array(w425) -> (w426:dbl[])
          n194 = call <vilib>:"Interpolate 1D.vi"("xi"=w426, "X"=w428, "Y"=w427) -> ("yi"=w424:dbl[])  [unwired: 6 in, 2 out]
          n195 = Index Array(array=w424) -> (element=w423:dbl)  [unwired: 1 in]
          n196 = Equal?(x=w423, y=w422) -> ()  [unwired: 1 out]
        }
        n197 = Build Array (concatenate)(w413, nan ("array")) -> (w412:dbl[])
        n198 = Build Array (concatenate)(w410, nan ("array")) -> (w409:dbl[])
      }
      n199 = for {
        tunnel: w398 -> [w477]
        tunnel: w401 -> [w475] mode=indexing
        tunnel: [w476] -> w402 mode=indexing
        n200 = Bundle("Relative Times NaN'd"=w477, w475) -> (w476:cluster{"Relative Times NaN'd":dbl[], dbl[]})  [unwired: 1 in]
      }
      "Compare Different Models vs TIME/DOSAGE" <- w402
      n201 = Delete From Array(array=w346, length=2) -> (array with subset deleted=w345:dbl[])  [unwired: 1 in, 1 out]
      n202 = for {
        tunnel: w400 -> [w471]
        tunnel: w404 -> [w469] mode=indexing
        tunnel: [w470] -> w406 mode=indexing
        n203 = Bundle("Relative Times NaN'd"=w471, w469) -> (w470:cluster{"Relative Times NaN'd":dbl[], dbl[]})  [unwired: 1 in]
      }
      "Ic and Temperature vs Time" <- w406
      n204 = Bundle(w359, w360) -> (→"Ic Power Law vs Time (COMPARE) 2":cluster{dbl[], waveform(dbl)[]})  [unwired: 1 in]
      n205 = for {
        tunnel: w349 -> [w474]
        tunnel: w403 -> [w472] mode=indexing
        tunnel: [w473] -> w355 mode=indexing
        n206 = Bundle("Relative Times NaN'd"=w474, w472) -> (w473:cluster{"Relative Times NaN'd":dbl[], dbl[]})  [unwired: 1 in]
      }
      n207 = Bundle("Relative Times NaN'd"=w400, w345) -> (w350:cluster{"Relative Times NaN'd":dbl[], dbl[]})  [unwired: 1 in]
      "Mean Run Temperature vs Time" <- w350
      n208 = call-poly <vilib>:"TSA Deviation and Variance.vi"("Xt"=w360) -> ()  [unwired: 7 in, 4 out]
      n209 = call "NEWTempInterpolate.vi"("method"=w367, "Ic Arr (Baseline 1st)"=w366, "Experimental Temp"=w346) -> ("Temp Data"=w374:dbl[], "Ic Data"=w382:dbl[], "xi used"=w368:dbl[], "Predicted Temp (C)"=w365:dbl[])  [unwired: 4 in, 1 out]
      n210 = for {
        tunnel: w340 -> [w437] mode=indexing
        tunnel: w378 -> [w436] mode=indexing
        tunnel: [w435] -> w377 mode=indexing
        tunnel: [w434] -> w358 mode=concatenating
        tunnel: [w433] -> w357 mode=concatenating
        n211 = Unbundle By Name(w436) -> ("Mean Temp Array"=w434:dbl[])
        n212 = Unbundle By Name(w437) -> ("Ic array (Power Law)"=w433:dbl[])
        n213 = Bundle("Mean Temp Array"=w434, "Ic array (Power Law)"=w433) -> (w435:T13)  [unwired: 1 in]
      }
      n214 = call "TempInterpolate.vi"("method"="TempInterpolate Method", "(Baseline 1st) Shifted"=w346, "True Experimental Data"=w366) -> ("Corrected Ic"=w372:dbl[])  [unwired: 3 in, 5 out]
      n215 = call "TempInterpolate - Reverse.vi"("method"="TempInterpolate Reverse Method", "Ic Arr (Baseline 1st)"=w366, "Experimental Temp"=w346) -> ("Corrected Temps"=w383:dbl[])  [unwired: 4 in, 4 out]
      n216 = call "KtoC.vi"("K"=w374) -> ("C"=w373:dbl[])  [unwired: 10 in]
      n217 = Bundle("C"=w373, "Ic Data"=w382) -> (w375:cluster{"C":dbl[], "Ic Data":dbl[]})  [unwired: 1 in]
      n218 = Bundle("Predicted Temp (C)"=w365, "xi used"=w368) -> (w369:T14)  [unwired: 1 in]
      n219 = Bundle("Relative Times NaN'd"=w349, "Corrected Ic"=w372) -> (w394:T15)  [unwired: 1 in]
      n220 = call <vilib>:"Interpolate 1D.vi"("xi"=w333, "X"=w335, "Y"=w334) -> ("yi"=w331:dbl[])  [unwired: 6 in, 2 out]
      n221 = Bundle("Relative Times NaN'd"=w349, "Corrected Temps"=w383) -> ()  [unwired: 1 in, 1 out]
      n222 = Build Array(w375, w369) -> (→"Ic Temperature Curve of THEVA HTS Tape 2":T16)
      n223 = Bundle(w346, "Corrected Ic"=w372) -> (w371:cluster{dbl[], "Corrected Ic":dbl[]})  [unwired: 1 in]
      n224 = Build Array (concatenate)(w377, w371) -> (→"Temperature vs Ic":T17)
      n225 = Bundle("yi"=w331, w330) -> (→"Dosage vs Ic":cluster{"yi":dbl[], dbl[]})  [unwired: 1 in]
      n226 = Bundle("Relative Times NaN'd"=w349, "Predicted Temp (C)"=w365) -> (w364:T18)  [unwired: 1 in]
      n227 = call "TempInterpolate.vi"("(Baseline 1st) Shifted"=w358) -> ("Raw Interpolated Ic"=w356:dbl[])  [unwired: 5 in, 5 out]
      n228 = Index Array(array=w356, index=0) -> (element=w352:dbl)
      n229 = Divide(x=w357, y=w356) -> (x/y=w351:dbl[])
      n230 = Multiply(x=w351, y=w352) -> (x*y=w348:dbl[])
      n231 = Delete From Array(array=w348) -> (array with subset deleted=w347:dbl[])  [unwired: 2 in, 1 out]
      n232 = Bundle("Relative Times NaN'd"=w349, w347) -> (w353:cluster{"Relative Times NaN'd":dbl[], dbl[]})  [unwired: 1 in]
      "Voltage @ 1st Current Increment" <- w329
    }
    frame #2 {
      n233 = Build Array (concatenate)(w500, w499, w498, w498) -> (→"Concatenated Ic vs Time":T19)
      n234 = Build Array (concatenate)(w492, w490, w491) -> (→"Temperature Normaliser":cluster{"Relative Times NaN'd":dbl[], dbl[]}[])
      n235 = Build Array (concatenate)(w503, w502, w490, w494) -> (→"Experimental Ic vs Temperature Corrected Ic":T20)
      n236 = Array Size(array=w489) -> (size(s)=w488:i32)
      n237 = for {
        N -> [w511]
        tunnel: w496 -> [w513] mode=indexing
        tunnel: w489 -> [w512] mode=indexing
        tunnel: [w511] -> w497
        tunnel: u32[] [16711930, 35095, 16860, 16748562, 16711680] ("Plot.Plot Color") -> [w506] mode=indexing
        n238 = property on="Ic Power Law vs Time (COMPARE)" class="XYGraph (strict)"("Active Plot"=w513, "Plot.Plot Name"=w512) -> ()  [unwired: 2 in, 2 out]
        n239 = property on="Concatenated Ic vs Time" class="XYGraph (strict)"("Active Plot"=w513, "Plot.Plot Name"=w512, "Plot.YScaleIdx"=u32 0 ("Plot.Y Scale Index"), "Plot.Point Style"=u8 5, "Plot.Line Width"=u8 1, "Plot.Plot Color"=w506, "Plot.Fill/Pt. Color"=w506, "Plot.Plot Interpolation"=u8 2, "Plot.Fill To"=i16 -1) -> ()  [unwired: 2 in, 2 out]
      }
      "NumPlots" <- w497
      n240 = property on="Ic Power Law vs Time (COMPARE)" class="XYGraph (strict)"("LegNumRows"=w488) -> ()  [unwired: 2 in, 2 out]
    }
    frame #3 {
      w537 = u32 1 ("Plot.Y Scale Index")
      w554 = u32 16448250 ("Plot.Plot Color")
      n241 = local read "NumPlots"() -> (w520:i32)
      n242 = Decrement(x=w537) -> (x-1=w538:u32)
      n243 = for {
        tunnel: u8[] [0, 2] ("Plot.Bar Plot Style") -> [w576] mode=indexing
        n244 = property on="Experimental Ic vs Temperature Corrected Ic" class="XYGraph (strict)"("Active Plot"=w576, "Plot.YScaleIdx"=u32 0 ("Plot.Y Scale Index")) -> ()  [unwired: 2 in, 2 out]
      }
      n245 = for {
        tunnel: u8[] [1, 3, 4, 5] ("Plot.Bar Plot Style") -> [w573] mode=indexing
        n246 = property on="Experimental Ic vs Temperature Corrected Ic" class="XYGraph (strict)"("Active Plot"=w573, "Plot.YScaleIdx"=u32 1 ("Plot.Y Scale Index")) -> ()  [unwired: 2 in, 2 out]
      }
      n247 = for {
        tunnel: u8[] [0, 1] ("Plot.Bar Plot Style") -> [w569] mode=indexing
        n248 = property on="Temperature Normaliser" class="XYGraph (strict)"("Active Plot"=w569, "Plot.YScaleIdx"=u32 0 ("Plot.Y Scale Index")) -> ()  [unwired: 2 in, 2 out]
      }
      n249 = property on="Dosage Characteristics" class="XYGraph (strict)"("Active Plot"=w537, "Plot.YScaleIdx"=u32 1 ("Plot.Y Scale Index"), "Plot.Plot Color"=u32 16754688, "Plot.Plot Name"="Cumulative", "YScale.ScaleFit"=u8 0 ("Y Scale.Scale Fit"), "Plot.Plot Interpolation"=u8 2, "Plot.Line Width"=u8 3) -> ()  [unwired: 2 in, 2 out]
      n250 = property on="Dosage Characteristics" class="XYGraph (strict)"("Active Plot"=w538, "Plot.YScaleIdx"=u32 0 ("Plot.Y Scale Index"), "Plot.Plot Color"=u32 16734720, "Plot.Plot Name"="Instantaneous", "YScale.ScaleFit"=u8 1 ("Y Scale.Scale Fit"), "Plot.Plot Interpolation"=u8 2, "Plot.Line Width"=u8 2, "LegNumRows"=u32 2 ("y")) -> ()  [unwired: 2 in, 2 out]
      n251 = Increment(x=w520) -> (x+1=w519:i32)
      n252 = Increment(x=w519) -> (x+1=w564:i32)
      n253 = property on="Concatenated Ic vs Time" class="XYGraph (strict)"("Active Plot"=w519, "Plot.YScaleIdx"=u32 1 ("Plot.Y Scale Index"), "Plot.Point Style"=u8 2, "Plot.Plot Color"=u32 16776770, "Plot.Plot Name"="Critical Points", "LegNumRows"=w564, "YScale.ScaleFit"=u8 0 ("Y Scale.Scale Fit"), "Plot.Plot Interpolation"=u8 0, "Plot.Line Width"=u8 2, "Plot.Bar Plot Style"=u8 1, "Plot.Fill To"=i16 -4, "Plot.Fill/Pt. Color"=w554) -> ()  [unwired: 2 in, 2 out]
      n254 = property on="Concatenated Ic vs Time" class="XYGraph (strict)"("Active Plot"=w520, "Plot.YScaleIdx"=u32 1 ("Plot.Y Scale Index"), "Plot.Point Style"=u8 0, "Plot.Plot Color"=u32 16734720, "Plot.Plot Name"="Cumulative Dosage", "Plot.Plot Interpolation"=u8 2, "Plot.Fill To"=i16 -1, "Plot.Line Width"=u8 2) -> ()  [unwired: 2 in, 2 out]
      n255 = for {
        tunnel: u8[] [2] ("Plot.Bar Plot Style") -> [w567] mode=indexing
        n256 = property on="Temperature Normaliser" class="XYGraph (strict)"("Active Plot"=w567, "Plot.YScaleIdx"=u32 1 ("Plot.Y Scale Index")) -> ()  [unwired: 2 in, 2 out]
      }
      n257 = property on="Experimental Ic vs Temperature Corrected Ic" class="XYGraph (strict)"("YScale.Maximum"=-200.4 ("Plot.Y Scale Index"), "YScale.Minimum"=-200.8 ("Plot.Y Scale Index"), "ActYScl"=0 ("Active Y Scale")) -> ()  [unwired: 2 in, 2 out]
      n258 = disable-structure shown="Enabled" {
        frame Enabled {
          n259 = property on="Experimental Ic vs Temperature Corrected Ic" class="XYGraph (strict)"("YScale.Maximum"=18.6 ("Plot.Y Scale Index"), "YScale.Minimum"=18.15 ("Plot.Y Scale Index"), "ActYScl"=1 ("Active Y Scale")) -> ()  [unwired: 2 in, 2 out]
        }
        frame Disabled {
        }
      }
      n260 = Increment(x=w519) -> (x+1=w565:i32)
      n261 = property on="Concatenated Ic vs Time" class="XYGraph (strict)"("Active Plot"=w565, "Plot.YScaleIdx"=u32 1 ("Plot.Y Scale Index"), "Plot.Point Style"=u8 2, "Plot.Plot Color"=u32 16776770, "Plot.Plot Name"="Critical Points", "YScale.ScaleFit"=u8 0 ("Y Scale.Scale Fit"), "Plot.Plot Interpolation"=u8 0, "Plot.Line Width"=u8 2, "Plot.Bar Plot Style"=u8 1, "Plot.Fill To"=i16 -3, "Plot.Fill/Pt. Color"=w554) -> ()  [unwired: 2 in, 2 out]
    }
  }
